vi "Get 2-variable Formula String Dialog.vi"(8 "error in (no error)":errorcluster, 10 "Variables":string="x, y", 11 "Formula Names":string) -> (0 "error out":errorcluster, 1 "Cancelled?":bool, 3 "Formula":string[](array[string]))   [LabVIEW 2021, in "GUI.lvlib"]
doc: "Displays a standard dialog box that prompts users to enter information, such as a user name and password.\n--------------------\n\nThis Express VI is configured as follows:\n\nMessage to Display to the User:\nThe inputs are: \nText Entry Box: Formula"
uses:
  GUI.lvlib
panel:
  in  "Formula(s)":string caption="x';y' ="
  out "String":string="Enter formula using x as variable (e.g.: 3.0*x**2 - 4.32):"
  in  "Cancel":bool
  in  "OK":bool caption="OK2"
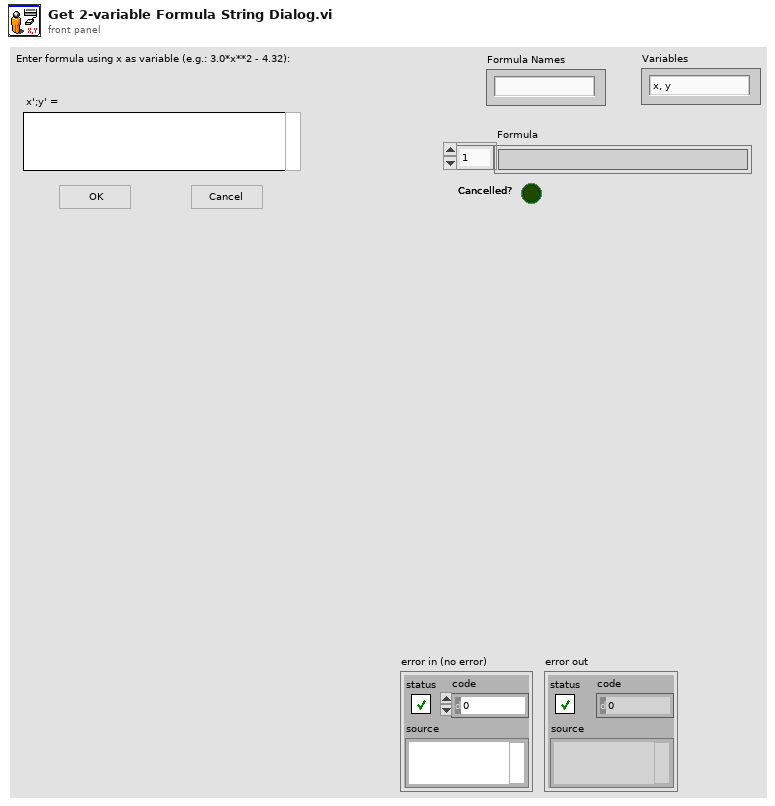
[diagram p1: front panel]
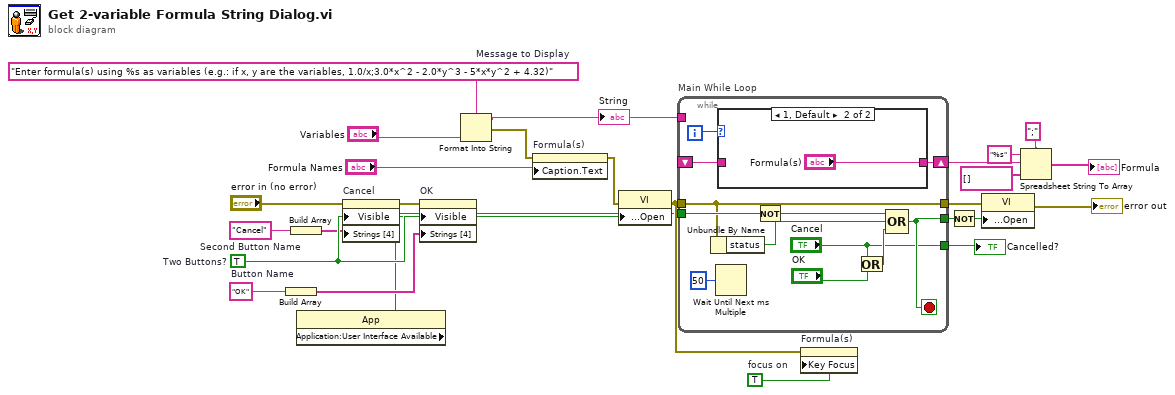
[diagram p0: block diagram]
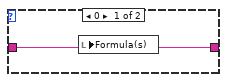
[diagram p2: hidden frame]
diagram:
  w14 = TRUE  # focus on
  w21 = "Cancel"  # Second Button Name
  w19 = "OK"  # Button Name
  w5 = "Enter formula(s) using %s as variables (e.g.: if x, y are the variables, 1.0/x;3.0*x^2 - 2.0*y^3 - 5*x*y^2 + 4.32)"  # Message to Display
  w26 = TRUE  # Two Buttons?
  n1 = Build Array(w19) -> (w20:string[])
  n2 = Build Array(w21) -> (w22:string[])
  n3 = property class="App"() -> ("Application:User Interface Available"=w13:bool)  [unwired: 2 in, 2 out]
  n4 = property on="Cancel" class="Bool"(error in="error in (no error)", "Visible"=w26, "Strings [4]"=w22) -> (error out=w25:errorcluster)  [unwired: 1 in, 1 out]
  n5 = property on="OK" class="Bool"(error in=w25, "Visible"=w26, "Strings [4]"=w20) -> ()  [unwired: 1 in, 2 out]
  n6 = Format Into String(format string=w5, "Variables") -> (resulting string=w6:string, error out=w2:errorcluster)  [unwired: 2 in]
  "String" <- w6
  n7 = property on="Formula(s)" class="Str"(error in=w2, "Caption.Text"="Formula Names") -> (error out=w1:errorcluster)  [unwired: 1 in, 1 out]
  n8 = property class="VI"(error in=w1, "Front Panel Window:Open"=w13) -> (error out=w18:errorcluster)  [unwired: 1 in, 1 out]
  n9 = while "Main While Loop" {
    tunnel: w13 -> [w37]
    tunnel: [w35] -> w23
    tunnel: w18 -> [w34]
    tunnel: [w34] -> w16
    tunnel: ["Cancel"] -> w12
    shift-right: [w28] -> w10
    shift-left: _ -> [w27]
    tunnel: w6 -> [_]
    i -> [w29]
    stop <- w35 stop-if-true
    n10 = Unbundle By Name(w34) -> ("status"=w32:bool)
    n11 = Wait Until Next ms Multiple(millisecond multiple=u32 50) -> ()  [unwired: 1 out]
    n12 = case shown="1, Default" w29 {
      tunnel: [w39 "Formula(s)"] -> w28
      tunnel: w27 -> [w39 _]
      frame 0 {
        n13 = local write "Formula(s)"(w39) -> ()
      }
      frame 1, Default {
      }
    }
    n14 = Not(x=w37) -> (.not. x?=w36:bool)
    n15 = Or(x="Cancel", y="OK") -> (x .or. y?=w33:bool)
    n16 = Compound Arithmetic op=OR(w36, w32, w33) -> (w35:bool)
  }
  "Cancelled?" <- w12
  n17 = property on="Formula(s)" class="Str"(error in=w18, "Key Focus"=w14) -> ()  [unwired: 1 in, 2 out]
  n18 = Not(x=w23) -> (.not. x?=w24:bool)
  n19 = property class="VI"(error in=w16, "Front Panel Window:Open"=w24) -> (error out=→"error out":errorcluster)  [unwired: 1 in, 1 out]
  n20 = Spreadsheet String To Array(delimiter (Tab)=";" ("search string"), format string="%s", spreadsheet string=w10, array type (2D Dbl)=string[] [] ("Formula")) -> (array=→"Formula":string[])
